vi "SYST_COMM_GPIB_RDEV_WBIN.vi"(0 "VISA IN":refnum<visa-resource-name>, 1 "BinBlk":string, 5 "error in":errorcluster, 7 "ID":i32) -> (14 "VISA Out":refnum<visa-resource-name>, 19 "error out":errorcluster)   [LabVIEW 2018, in "PNA-X.lvlib"]
doc: "SYSTem:COMMunicate:GPIB:RDEVice:WBINary <ID>,<data> \n(Write-only) Sends data to a GPIB pass-through device. This command requires a header that \nspecifies the size of the data to be written. The header (described below) is not passed along to the \ndevice. \nUse this command if too many embedded quotes prevent you from using \nSYST:COMM:GPIB:RDEV:WRIT. \nUse SYST:COMM:GPIB:RDEV:OPEN to open the pass through session. \nParameters \n<ID> Session identification number that was returned with the OPEN? command. \n<data> Data to be sent to the GPIB pass-through device. Use the following syntax: \n#<num digits><byte count><data bytes><NL><END> \n<num_digits> specifies how many digits are contained in <byte_count> \n<byte_count> specifies how many data bytes will follow in <data bytes> \nExamples SYSTem:COMMunicate:GPIB:RDEVice:WBINary 101,#17ABC+XYZ<nl><end> \n# - always sent before data.\n1871\n\n1 - specifies that the byte count is one digit (7). \n7 - specifies the number of data bytes that will follow, not counting \n<NL><END>. \nABC+XYZ - Data block \n<nl><end> - always sent at the end of block data. \nThe following example sends a line feed at the end. \nSYST:COMM:GPIB:RDEV:WBIN 1,#210SYST:PRES<EOL> \nThe <EOL> represents your linefeed character. \nQuery Syntax Not Applicable \nDefault Not Applicable"
uses:
  PNA-X.lvlib
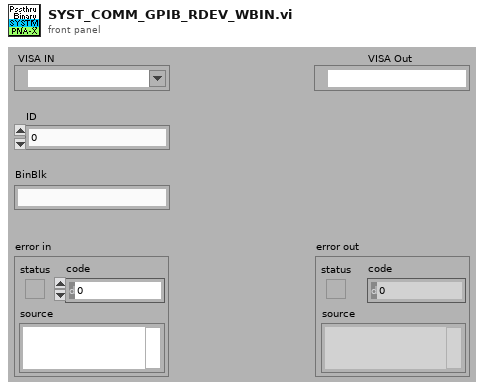
[diagram p1: front panel]
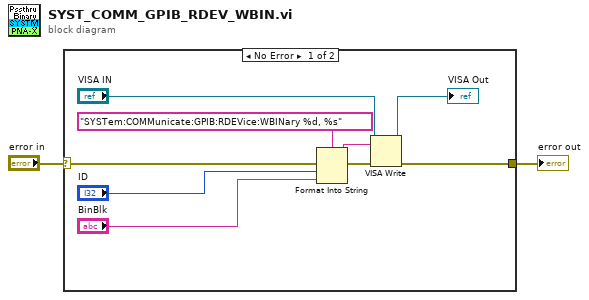
[diagram p0: block diagram]
diagram:
  n1 = case shown="No Error" "error in" {
    selector: "error in" -> [w11 w12]
    tunnel: [w6 w12] -> w1
    frame No Error {
      n2 = Format Into String(format string="SYSTem:COMMunicate:GPIB:RDEVice:WBINary %d, %s" ("Cmdline"), error in=w11, "ID", "BinBlk") -> (resulting string=w9:string, error out=w10:errorcluster)  [unwired: 1 in]
      n3 = VISA Write(VISA resource name="VISA IN", write buffer=w9, error in (no error)=w10) -> (VISA resource name out=→"VISA Out":refnum<visa-resource-name>, error out=w6:errorcluster)  [unwired: 1 out]
    }
    frame Error {
    }
  }
  "error out" <- w1
